vi "Read Caller SubPanel.vi"(8 "error in (no error)":errorcluster, 11 "Coins in":refnum<class "Coins.lvclass">) -> (0 "error out":errorcluster, 2 "Caller SubPanel":refnum<vi>, 3 "Coins out":refnum<class "Coins.lvclass">)   [LabVIEW 2020, in "Coins.lvlib" / "Coins.lvclass"]
uses:
  Coins.lvclass
  Coins.lvclass/Coins.ctl
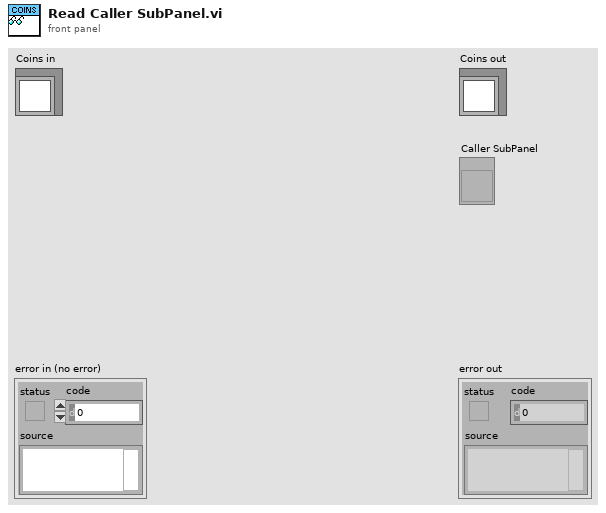
[diagram p1: front panel]
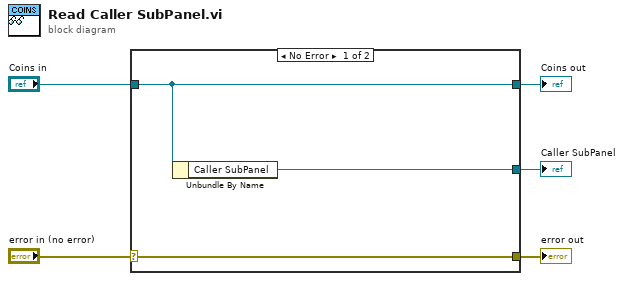
[diagram p0: block diagram]
diagram:
  n1 = case shown="No Error" "error in (no error)" {
    selector: "error in (no error)" -> [w8 w9]
    tunnel: [w8 w9] -> w4
    tunnel: [w7 w10] -> w2
    tunnel: "Coins in" -> [w7 w10]
    tunnel: [w6 _] -> w1
    frame No Error {
      n2 = Unbundle By Name(w7) -> ("Caller SubPanel"=w6:refnum<vi>)
    }
    frame Error {
    }
  }
  "error out" <- w4
  "Coins out" <- w2
  "Caller SubPanel" <- w1
